vi "SetExposure.vi"(8 "error in (no error)":errorcluster, 10 "Exposure(ms)":u32=10000, 11 "ZWO_ASI in":refnum<class "ZWO_ASI.lvclass">) -> (0 "error out":errorcluster, 3 "ZWO_ASI out":refnum<class "ZWO_ASI.lvclass">)   [LabVIEW 2023, in "ZWO_ASI.lvlib" / "ZWO_ASI.lvclass"]
uses:
  ZWO_ASI.lvclass
  Labview_ASI_demo_64bit_221128/user.lib/ASICamera2_no_err/ASICamera2_no_err.lvlib
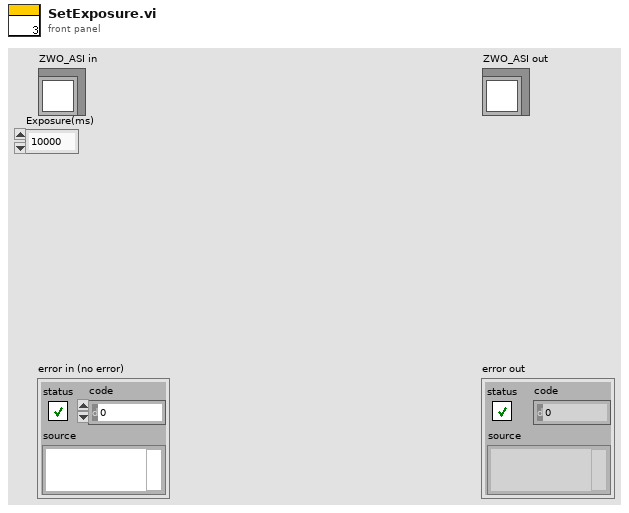
[diagram p1: front panel]
types:
  T1 = cluster{"name":string, "ControlType":u32, "plValue out":i32, "MaxValue":i32, "MinValue":i32}[]
  T2 = cluster{"name":string, "ControlType":u32, "plValue out":i32, "MaxValue":i32, "MinValue":i32}
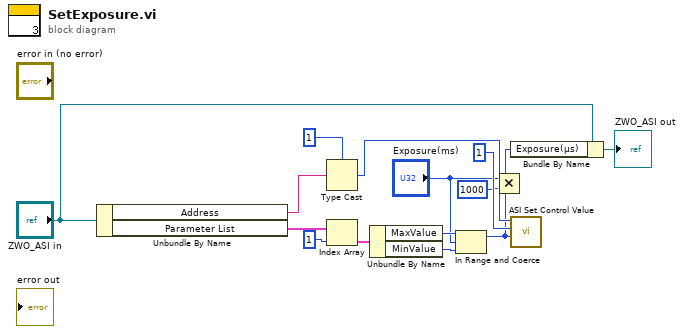
[diagram p0: block diagram]
diagram:
  n1 = Unbundle By Name("ZWO_ASI in") -> ("Address"=w7:string, "Parameter List"=w12:T1)
  n2 = Type Cast(type=1 ("ControlType"), x=w7) -> (*(type *) &x=w6:i32)
  n3 = Index Array(array=w12, index=1) -> (element=w10:T2)
  n4 = Unbundle By Name(w10) -> ("MaxValue"=w9:i32, "MinValue"=w8:i32)
  n5 = In Range and Coerce(upper limit=w9, x="Exposure(ms)", lower limit=w8) -> (coerced(x)=w3:u32)  [unwired: 1 out]
  n6 = Multiply(x="Exposure(ms)", y=u32 1000) -> ()  [unwired: 1 out]
  n7 = Bundle By Name(cluster="ZWO_ASI in", "Exposure(μs)"=w3) -> (→"ZWO_ASI out":refnum<class "ZWO_ASI.lvclass">)
  n8 = call "ASI Set Control Value.vi"("lValue"=w3, "ControlType"=1, "iCameraID"=w6) -> ()  [unwired: 8 in, 1 out]
